vi "ATF-Pump-AI V Start.vi"(8 "error in":errorcluster, 9 "AI V":T1(array[cluster]), 11 "Refnum in":refnum<k21>) -> (0 "error out":errorcluster, 3 "Refnum out":refnum<k21>)   [LabVIEW 2022 SP3]
doc: "This VI is for start for Analog voltage Start task"
uses:
  <vilib>/DAQmx/configure/timing.llb/DAQmx Timing (Sample Clock).vi
  <vilib>/DAQmx/configure/trigger.llb/DAQmx Start Trigger (Digital Edge).vi
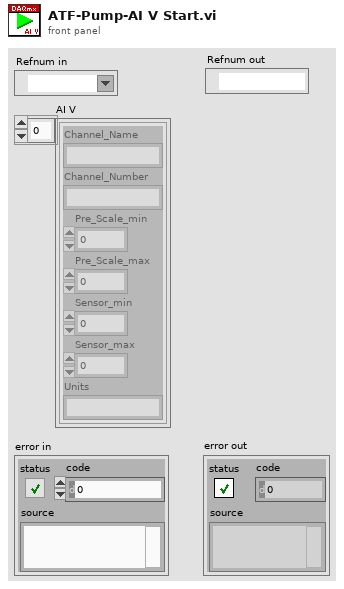
[diagram p1: front panel]
types:
  T1 = cluster{"Channel_Name":string, "Channel_Number":string, "Pre_Scale_min":dbl, "Pre_Scale_max":dbl, "Sensor_min":dbl, "Sensor_max":dbl, "Units":string}[]
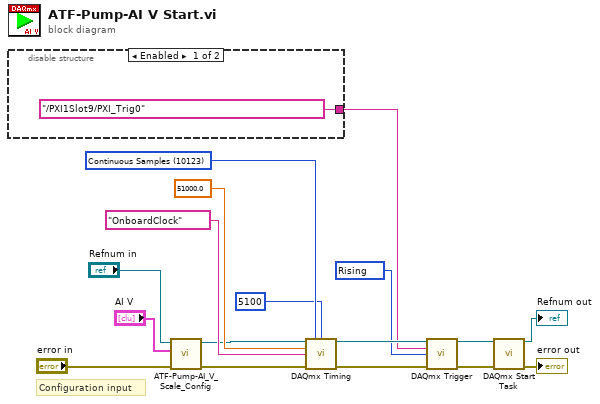
[diagram p0: block diagram]
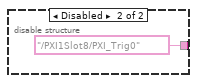
[diagram p2: hidden frame]
diagram:
  w13 = 10280 items=["Rising"=10280, "Falling"=10171] ("edge")
  w10 = 10123 items=["Finite Samples"=10178, "Continuous Samples"=10123, "Hardware Timed Single Point"=12522] ("sample mode")
  # "Configuration input"
  n1 = disable-structure shown="Enabled" {
    disable-tunnel: [tag "/PXI1Slot9/PXI_Trig0" ("source") tag "/PXI1Slot8/PXI_Trig0" ("source")] -> w1
    frame Enabled {
    }
    frame Disabled {
    }
  }
  n2 = call "ATF-Pump-AI_V_Scale_Config.vi"("error in"="error in", "AI C"="AI V", "task in"="Refnum in") -> ("error out"=w3:errorcluster, "task out"=w8:refnum<k21>)  [unwired: 7 in]
  n3 = call-poly <vilib>:"DAQmx Timing.vi"("task/channels in"=w8, "sample mode"=w10, "samples per channel"=5100, "rate"=51000.0, "source"=tag "OnboardClock", "error in"=w3) -> ("task out"=w14:refnum<k21>, "error out"=w6:errorcluster)  [unwired: 8 in]
  n4 = call-poly <vilib>:"DAQmx Trigger.vi"("task/channels in"=w14, "source"=w1, "edge"=w13, "error in"=w6) -> ("task out"=w16:refnum<k21>, "error out"=w15:errorcluster)  [unwired: 10 in]
  n5 = call <vilib>:"DAQmx Start Task.vi"("task/channels in"=w16, "error in"=w15) -> ("task out"=→"Refnum out":refnum<k21>, "error out"=→"error out":errorcluster)  [unwired: 12 in]
